vi "Find Log File.vi"(8 "error in (no error)":errorcluster, 11 "Root Path":path) -> (0 "error out":errorcluster, 3 "Log Data":string[][](array[string]))   [LabVIEW 2014]
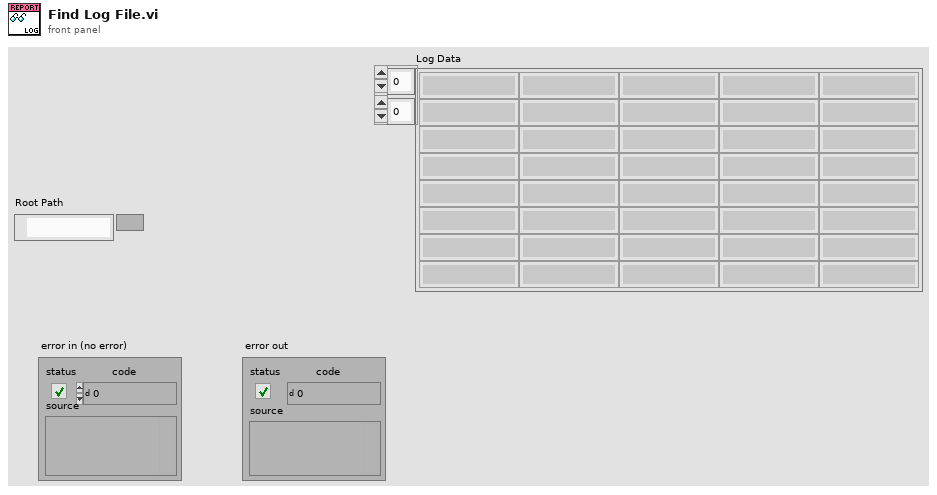
[diagram p1: front panel]
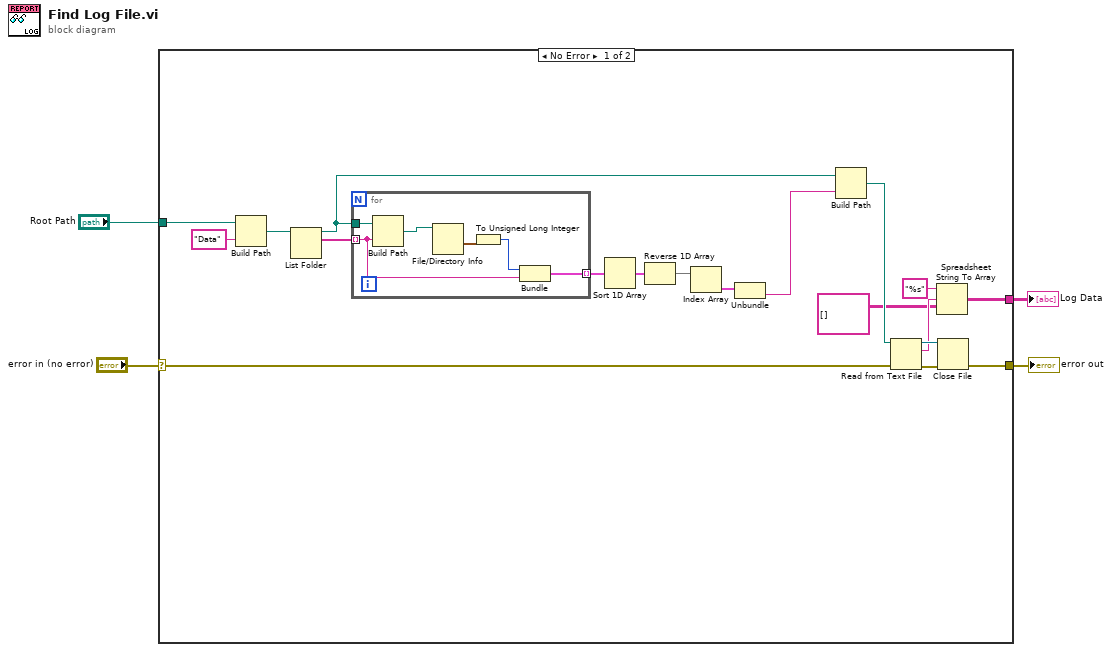
[diagram p0: block diagram]
diagram:
  n1 = case shown="No Error" "error in (no error)" {
    selector: "error in (no error)" -> [w20 w30]
    tunnel: "Root Path" -> [w23 _]
    tunnel: [w21 w30] -> w3
    tunnel: [w19 _] -> w1
    frame No Error {
      n2 = Build Path(base path=w23, name or relative path="Data") -> (appended path=w10:path)
      n3 = List Folder(path=w10) -> (path out=w5:path, filenames=w12:string[])  [unwired: 3 in, 2 out]
      n4 = for {
        tunnel: w12 -> [w25] mode=indexing
        tunnel: w5 -> [w29]
        tunnel: [w27] -> w11 mode=indexing
        n5 = Build Path(base path=w29, name or relative path=w25) -> (appended path=w26:path)
        n6 = File/Directory Info(path=w26) -> (last mod=w24:timestamp)  [unwired: 1 in, 6 out]
        n7 = To Unsigned Long Integer(number=w24) -> (unsigned 32bit integer=w28:u32)
        n8 = Bundle(w28, w25) -> (w27:cluster{u32, string})  [unwired: 1 in]
      }
      n9 = Sort 1D Array(array=w11) -> (sorted array=w9:cluster{u32, string}[])
      n10 = Reverse 1D Array(array=w9) -> (reversed array=w8:cluster{u32, string}[])
      n11 = Index Array(array=w8) -> (element=w7:cluster{u32, string})  [unwired: 1 in]
      n12 = Unbundle(w7) -> (w6:string)  [unwired: 1 out]
      n13 = Build Path(base path=w5, name or relative path=w6) -> (appended path=w18:path)
      n14 = Read from Text File(file (use dialog)=w18, error in=w20) -> (refnum out=w16:refnum<file>, text=w15:string, error out=w17:errorcluster)  [unwired: 2 in, 1 out]
      n15 = Spreadsheet String To Array(format string="%s", spreadsheet string=w15, array type (2D Dbl)=string[][] []) -> (array=w19:string[][])  [unwired: 1 in]
      n16 = Close File(refnum=w16, error in=w17) -> (error out=w21:errorcluster)  [unwired: 1 out]
    }
    frame Error {
    }
  }
  "error out" <- w3
  "Log Data" <- w1
